vi "Read Coords.vi"(8 "error in (no error)":errorcluster, 11 "ControlMouseDownMsg in":refnum<class "ControlMouseDownMsg.lvclass">) -> (0 "error out":errorcluster, 2 "Coords":T1, 3 "ControlMouseDownMsg out":refnum<class "ControlMouseDownMsg.lvclass">)   [LabVIEW 2017, in "ActorEvents.lvlib" / "ControlMouseDownMsg.lvclass"]
uses:
  <vilib>/gpm_packages/@cs/mva-viewable/Source/ActorEvents/IEventAggregator Messages/ControlMouseDownMsg/ControlMouseDownMsg.lvclass
  <vilib>/Utility/miscctls.llb/LVPoint32TypeDef.ctl
  <vilib>/gpm_packages/@cs/mva-viewable/Source/ActorEvents/IEventAggregator Messages/ControlMouseDownMsg/ControlMouseDownMsg.lvclass/ControlMouseDownMsg.ctl
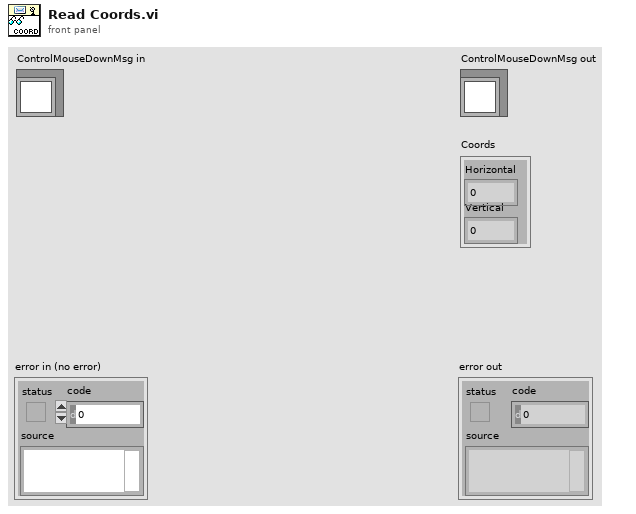
[diagram p1: front panel]
types:
  T1 = typedef "LVPoint32TypeDef.ctl" = cluster{"Horizontal":i32, "Vertical":i32}
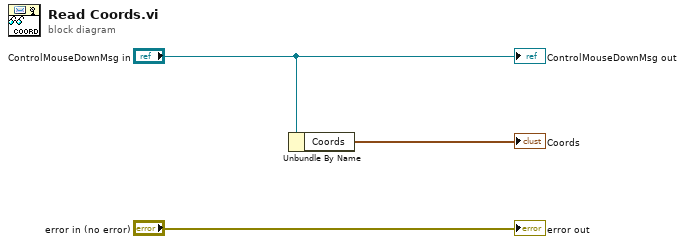
[diagram p0: block diagram]
diagram:
  n1 = Unbundle By Name("ControlMouseDownMsg in") -> ("Coords"=→"Coords":T1)
  "error out" <- "error in (no error)"
  "ControlMouseDownMsg out" <- "ControlMouseDownMsg in"
